vi "test3caller.vi"() -> ()   [LabVIEW 2012]
panel:
  in  "stop":bool
  in  "error in (no error)":errorcluster
  in  "Image Type":T1=7 items=["Grayscale (U8)", "Grayscale (I16)", "Grayscale (SGL)", "Complex (CSG)", "RGB (U32)", "HSL (U32)", "RGB (U64)", "Grayscale (U16)"]
  in  "Image Name":string="untitled"
  out "Image":T2(plugin-control)
  in  "fmt":T3(ring)
  in  "index":i32
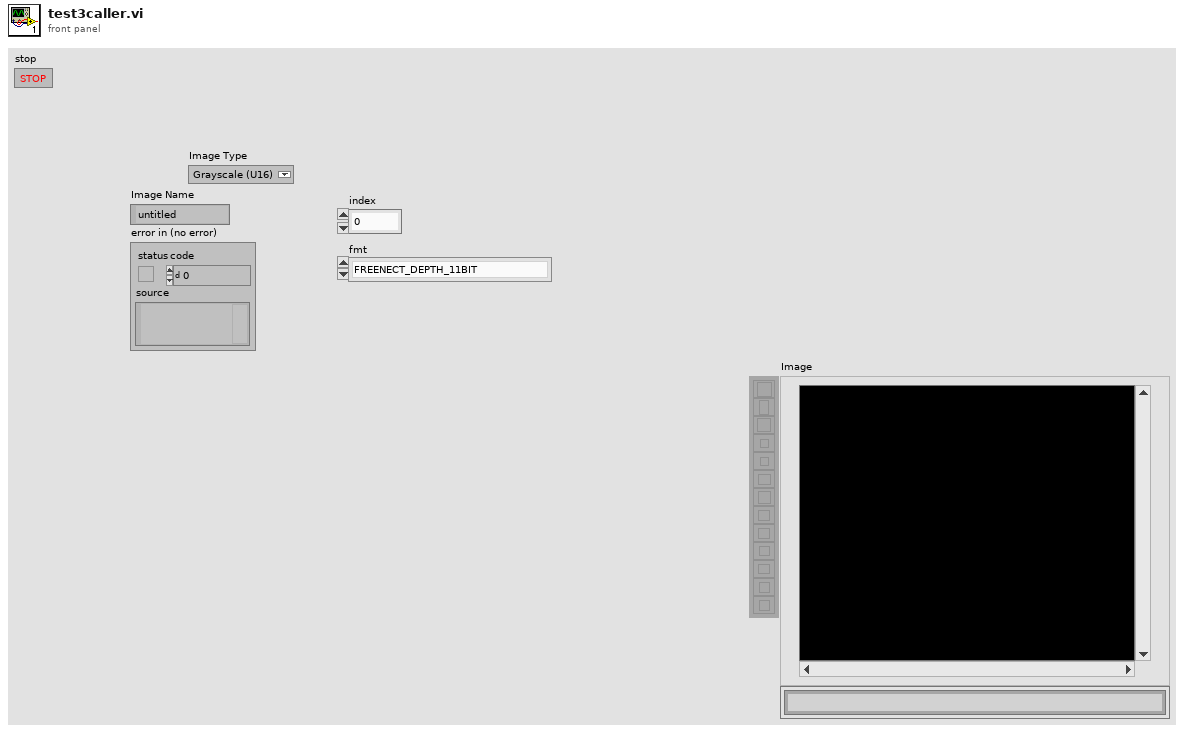
[diagram p1: front panel]
types:
  T1 = typedef "Image Type" = u32
  T2 = typedef "IMAQ Image.ctl" = refnum<image>
  T3 = enum16{"FREENECT_DEPTH_11BIT", "FREENECT_DEPTH_10BIT", "FREENECT_DEPTH_11BIT_PACKED", "FREENECT_DEPTH_10BIT_PACKED"}
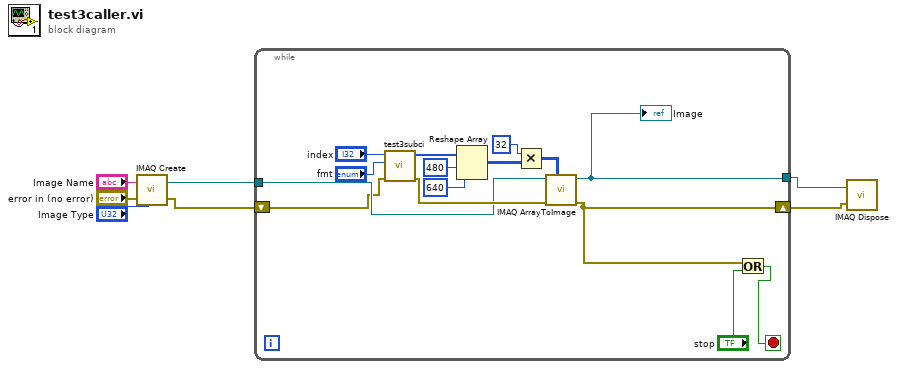
[diagram p0: block diagram]
diagram:
  n1 = call "IMAQ Create"("Image Name"="Image Name", "Image Type"="Image Type", "error in (no error)"="error in (no error)") -> ("New Image"=w4:T2, "error out"=w1:errorcluster)  [unwired: 2 in]
  n2 = while {
    tunnel: w4 -> [w13]
    tunnel: [w8] -> w3
    shift-right: [w11] -> w2
    shift-left: w1 -> [w12]
    stop <- w10 stop-if-true
    n3 = call "test3subci.vi"("error in (no error)"=w12, "fmt"="fmt", "index"="index") -> ("error out"=w17:errorcluster, "Destination"=w20:u16[])  [unwired: 7 in]
    n4 = Reshape Array(w20, 480 ("dimension size"), 640 ("dimension size")) -> (w16:u16[][])
    n5 = Multiply(x=32, y=w16) -> (x*y=w14:i32[][])
    n6 = call "IMAQ ArrayToImage"("Image Pixels (U16)"=w14, "error in (no error)"=w17, "Image"=w13) -> ("error out"=w11:errorcluster, "Image Out"=w8:T2)  [unwired: 3 in, 4 out]
    "Image" <- w8
    n7 = Or(x=w11, y="stop") -> (x .or. y?=w10:bool)
  }
  n8 = call "IMAQ Dispose"("Image"=w3, "error in (no error)"=w2) -> ()  [unwired: 4 in, 1 out]
